vi "to-matlab2.vi"() -> ()   [LabVIEW 2018]
uses:
  <vilib>/Platform/TimedLoop/XDataNode/timing_clust.ctl
  <vilib>/Platform/TimedLoop/XDataNode/nitl_modes.ctl
  <vilib>/Platform/TimedLoop/XDataNode/wakeup.ctl
  <vilib>/DAQmx/read.llb/DAQmx Read (Counter U32 1Chan 1Samp).vi
  <vilib>/DAQmx/read.llb/DAQmx Read (Analog 1D Wfm NChan NSamp).vi
  <extravilib>/ChannelInstances/Stream-u32/EndpointRead.vi
  <extravilib>/ChannelInstances/Stream-a[.](wfm(dbl))/EndpointRead.vi
  <extravilib>/ChannelInstances/Stream-u32/Endpoint.vi
  <extravilib>/ChannelInstances/Stream-a[.](wfm(dbl))/Endpoint.vi
  <vilib>/DAQmx/create/channels.llb/DAQmx Create Channel (AI-Voltage-Basic).vi
  <vilib>/DAQmx/configure/timing.llb/DAQmx Timing (Sample Clock).vi
  <vilib>/DAQmx/create/channels.llb/DAQmx Create Channel (CI-Count Edges).vi
  <extravilib>/ChannelInstances/Stream-a[.](wfm(dbl))/Instantiate.vi
  <extravilib>/ChannelInstances/Stream-a[.](wfm(dbl))/)Channel.vi
  <resource>/ChannelSupport/_ChannelSupport/WaitIfNeeded.vi
  <vilib>/DAQmx/miscellaneous.llb/DAQmx Fill In Error Info.vi
  <extravilib>/ChannelInstances/Stream-u32/Instantiate.vi
  <extravilib>/ChannelInstances/Stream-u32/)Channel.vi
  <vilib>/platform/TimedLoop/XDataNode/XDataNode.xnode
  <extravilib>/ChannelInstances/Stream-u32.lvlib
  <extravilib>/ChannelInstances/Stream-a[.](wfm(dbl)).lvlib
  <vilib>/Platform/TimedLoop/XDataNode/XDNodeRunTimeDep.lvlib
panel:
  in  "Reset Button":bool
  in  "Start Button":bool
  in  "Stop Button":bool
  in  "Settings Button":bool
  in  "Brake Torque":bool
  in  "Dynamometer\nRPM":bool
  in  "Batterycurrent":bool
  in  "Batteryvoltage":bool
  in  "All Graphs":bool
  out "Actual Start [i]":i64
  in  "Tab Control":enum32{"Graphs", "Settings"}(tab)
  out "Brake Torque":dynamicdata(graph)
  out "Battery Current":dynamicdata(graph)
  in  "STOP Measurements":bool
  out "Battery Voltage":dynamicdata(graph)
  out "Actual End [i-1]":i64
  in  "Refresh Rate in ms":u32=50
  in  "Sample Rate":dbl=1000.0 format="%0.2f"
  in  "Sample Mode":i32(ring)=10123 items=["Finite Samples"=10178, "Continuous Samples"=10123, "Hardware Timed Single Point"=12522]
  in  "Samples per Channel":i32=1000
  in  "AI Channel 3":tag="Dev1/ai2"
  in  "Name 3":string="M_brems"
  in  "Measurement Type 3":i32(ring)=10083 items=["Default"=-1, "RSE"=10083, "NRSE"=10078, "Differential"=10106, "Pseudodifferential"=12529]
  in  "AI Channel 2":tag="Dev1/ai1"
  in  "Name 2":string="I_batt"
  in  "Measurement Type 2":i32(ring)=10083 items=["Default"=-1, "RSE"=10083, "NRSE"=10078, "Differential"=10106, "Pseudodifferential"=12529]
  in  "AI Channel":tag="Dev1/ai0"
  in  "Name":string="U_batt"
  in  "Measurement Type":i32(ring)=-1 items=["Default"=-1, "RSE"=10083, "NRSE"=10078, "Differential"=10106, "Pseudodifferential"=12529]
  in  "Counter Channel":tag="Dev1/ctr0"
  in  "Counter Name":string="Counter"
  in  "Battery Current Scale":dbl=25.0
  in  "Battery Voltage Scale":dbl=9.97
  in  "Brake Torque Scale":dbl=1.0
  # "Sampling Options"
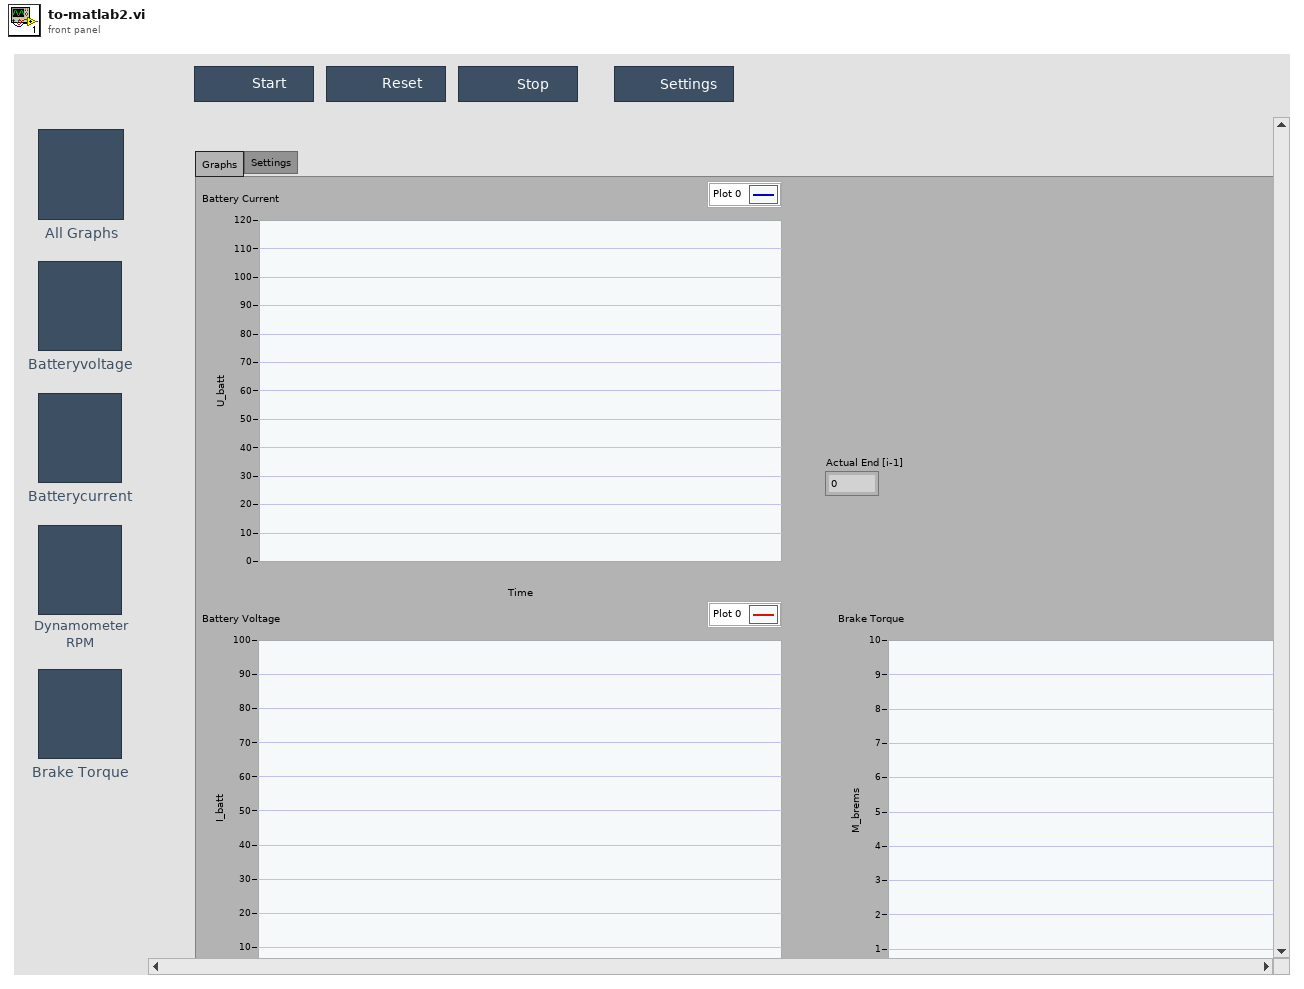
[diagram p1: front panel]
types:
  T1 = typedef "XDNodeRunTimeDep.lvlib/timing_clust.ctl" = cluster{"Expected End [f-1]":u64, "Actual End [f-1]":u64, "Finished Late? [f-1]":bool, "Expected End [i-1]":u64, "Actual End [i-1]":u64, "Finished Late? [i-1]":bool, "Expected Start [i]":u64, "Actual Start [i]":u64, "Expected Start [f]":u64, "Actual Start [f]":u64, "Source Name":string, "Structure Name":string, "Period":i64, "Deadline":i64, "Offset":i64, "Start":i64, "Priority":i32, "Timeout":i32, "Mode":T2, "Wakeup Reason":T3, "Error":errorcluster, "Source Type":string, "Secondary Source Type":string, "Global End Time":u64, "Global Start Time":u64, "Frame Duration":u64, "Iteration Duration":u64, "Assigned CPU":i32, "I/O Scan Engine Mode":u32}
  T2 = typedef "XDNodeRunTimeDep.lvlib/nitl_modes.ctl" = enum32{"No Change", "Process missed periods, maintain original phase", "Discard missed periods, maintain original phase", "Process missed periods, ignore original phase", "Discard missed periods, ignore original phase"}
  T3 = typedef "XDNodeRunTimeDep.lvlib/wakeup.ctl" = enum32{"Normal", "Aborted", "Asynchronous wakeup", "Timing source error", "Timed loop error", "Timeout"}
  T4 = typedef "Stream-u32.lvlib/)Channel.ctl" = refnum<queue>
  T5 = typedef "Stream-a[.](wfm(dbl)).lvlib/)Channel.ctl" = refnum<queue>
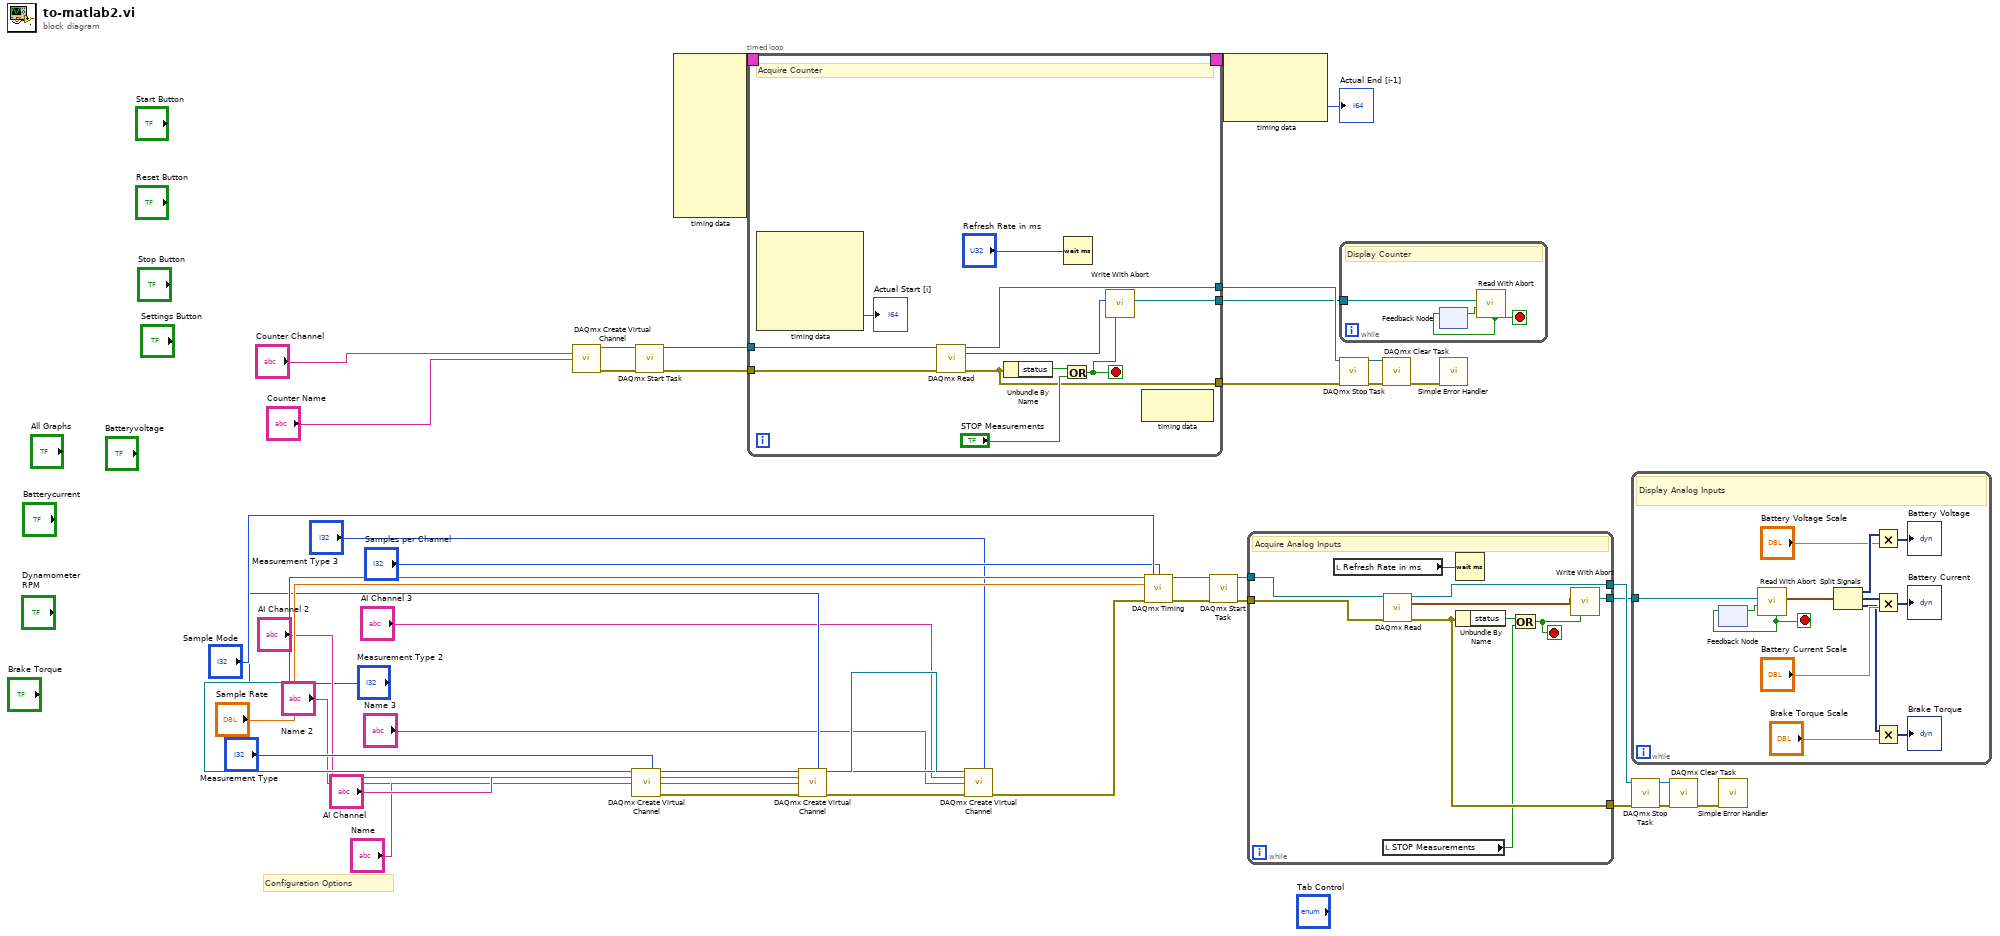
[diagram p0: block diagram]
diagram:
  # "Configuration Options"
  n1 = call-poly <vilib>:"DAQmx Create Virtual Channel.vi"("counter"="Counter Channel", "name to assign"="Counter Name") -> ("task out"=w43:refnum<k21>, "error out"=w42:errorcluster)  [unwired: 12 in]
  n2 = call-poly <vilib>:"DAQmx Create Virtual Channel.vi"("input terminal configuration"="Measurement Type", "physical channels"="AI Channel", "name to assign"="Name") -> ("task out"=w17:refnum<k21>, "error out"=w16:errorcluster)  [unwired: 11 in]
  n3 = call <vilib>:"DAQmx Start Task.vi"("task/channels in"=w43, "error in"=w42) -> ("task out"=w41:refnum<k21>, "error out"=w40:errorcluster)  [unwired: 12 in]
  n4 = node-c288() -> (w3:T1)  [unwired: 10 in]
  n5 = timed-loop {
    tunnel: w41 -> [w54]
    tunnel: w40 -> [w53]
    tunnel: [w50] -> w37
    tunnel: [w52] -> w36
    tunnel: [w46] -> w34
    timing: w3 -> [_]
    timing-out: [_] -> w2
    stop <- w47 stop-if-true
    # "Acquire Counter"
    n6 = node-c288() -> (→"Actual Start [i]":i64)  [unwired: 1 in, 5 out]
    n7 = call-poly <vilib>:"DAQmx Read.vi"("task/channels in"=w54, "error in"=w53) -> ("task out"=w52:refnum<k21>, "data"=w48:u32, "error out"=w50:errorcluster)  [unwired: 11 in]
    n8 = Unbundle By Name(w50) -> ("status"=w49:bool)
    n9 = Or(x=w49, y="STOP Measurements") -> (x .or. y?=w47:bool)
    n10 = Wait (ms)(milliseconds to wait="Refresh Rate in ms") -> ()  [unwired: 1 out]
    n11 = call <extravilib>:"Write With Abort.vi"("abort"=w47, "element"=w48) -> ("channel"=w46:T4)  [unwired: 6 in, 3 out]
    n12 = node-c288() -> ()  [unwired: 1 in, 1 out]
  }
  n13 = call-poly <vilib>:"DAQmx Create Virtual Channel.vi"("task in"=w17, "input terminal configuration"="Measurement Type 2", "physical channels"="AI Channel 2", "name to assign"="Name 2", "error in"=w16) -> ("task out"=w15:refnum<k21>, "error out"=w13:errorcluster)  [unwired: 9 in]
  n14 = call-poly <vilib>:"DAQmx Create Virtual Channel.vi"("task in"=w15, "input terminal configuration"="Measurement Type 3", "physical channels"="AI Channel 3", "name to assign"="Name 3", "error in"=w13) -> ("task out"=w14:refnum<k21>, "error out"=w12:errorcluster)  [unwired: 9 in]
  n15 = call-poly <vilib>:"DAQmx Timing.vi"("task/channels in"=w14, "sample mode"="Sample Mode", "samples per channel"="Samples per Channel", "rate"="Sample Rate", "error in"=w12) -> ("task out"=w30:refnum<k21>, "error out"=w29:errorcluster)  [unwired: 9 in]
  n16 = call <vilib>:"DAQmx Start Task.vi"("task/channels in"=w30, "error in"=w29) -> ("task out"=w21:refnum<k21>, "error out"=w20:errorcluster)  [unwired: 12 in]
  n17 = node-c288(w2) -> (→"Actual End [i-1]":i64)  [unwired: 2 out]
  n18 = while {
    tunnel: w21 -> [w67]
    tunnel: [w65] -> w28
    tunnel: [w66] -> w27
    tunnel: [w61] -> w24
    tunnel: w20 -> [w58]
    stop <- w62 stop-if-true
    # "Acquire Analog Inputs"
    n19 = local read "Refresh Rate in ms"() -> (w59:u32)
    n20 = local read "STOP Measurements"() -> (w60:bool)
    n21 = call-poly <vilib>:"DAQmx Read.vi"("task/channels in"=w67, "error in"=w58) -> ("task out"=w66:refnum<k21>, "data"=w63:waveform(dbl)[], "error out"=w65:errorcluster)  [unwired: 11 in]
    n22 = Wait (ms)(milliseconds to wait=w59) -> ()  [unwired: 1 out]
    n23 = Unbundle By Name(w65) -> ("status"=w64:bool)
    n24 = Or(x=w64, y=w60) -> (x .or. y?=w62:bool)
    n25 = call <extravilib>:"Write With Abort.vi"("abort"=w62, "element"=w63) -> ("channel"=w61:T5)  [unwired: 6 in, 3 out]
  }
  n26 = while {
    tunnel: w34 -> [w70]
    stop <- w68 stop-if-true
    # "Display Counter"
    n27 = feedback #1() -> (w69:bool)  [unwired: 1 in]
    n28 = call <extravilib>:"Read With Abort.vi"("abort"=w69, "channel"=w70) -> ("aborted?"=w68:bool)  [unwired: 4 in, 5 out]
    n29 = feedback-in #1(w68) -> ()
  }
  n30 = call <vilib>:"DAQmx Stop Task.vi"("task/channels in"=w36, "error in"=w37) -> ("task out"=w35:refnum<k21>, "error out"=w39:errorcluster)  [unwired: 12 in]
  n31 = call <vilib>:"DAQmx Clear Task.vi"("task in"=w35, "error in"=w39) -> ("error out"=w38:errorcluster)  [unwired: 13 in]
  n32 = call <vilib>:"Simple Error Handler.vi"("error in (no error)"=w38) -> ()  [unwired: 4 in, 5 out]
  n33 = while {
    tunnel: w24 -> [w83]
    stop <- w82 stop-if-true
    # "Display Analog Inputs"
    n34 = feedback #2() -> (w81:bool)  [unwired: 1 in]
    n35 = call <extravilib>:"Read With Abort.vi"("abort"=w81, "channel"=w83) -> ("element"=w80:waveform(dbl)[], "aborted?"=w82:bool)  [unwired: 4 in, 4 out]
    n36 = feedback-in #2(w82) -> ()
    n37 = Split Signals(w80) -> (w76:dynamicdata, w79:dynamicdata, w73:dynamicdata)  [unwired: 3 in]
    n38 = Multiply(x=w76, y="Battery Voltage Scale") -> (x*y=→"Battery Voltage":dynamicdata)
    n39 = Multiply(x=w79, y="Battery Current Scale") -> (x*y=→"Battery Current":dynamicdata)
    n40 = Multiply(x=w73, y="Brake Torque Scale") -> (x*y=→"Brake Torque":dynamicdata)
  }
  n41 = call <vilib>:"DAQmx Stop Task.vi"("task/channels in"=w27, "error in"=w28) -> ("task out"=w31:refnum<k21>, "error out"=w33:errorcluster)  [unwired: 12 in]
  n42 = call <vilib>:"DAQmx Clear Task.vi"("task in"=w31, "error in"=w33) -> ("error out"=w32:errorcluster)  [unwired: 13 in]
  n43 = call <vilib>:"Simple Error Handler.vi"("error in (no error)"=w32) -> ()  [unwired: 4 in, 5 out]
